vi "Shot Info Collection.vi"(6 "Vision Target Aligned? in":bool, 7 "Current Angle":dbl, 8 "Reinit?":bool, 9 "Shot Type":T1, 10 "Vision Packet":T2, 11 "Shooter Presets":T3={"Batter Shot"={"L"=0.0, "R"=0.0, "A"=0.0}, "Deep Middle"={"L"=0.0, "R"=0.0, "A"=0.0}, "Manual Shot"={"L"=0.0, "R"=0.0, "A"=0.0}, "Left Ticks Per Rotation"=0.0, "Right Ticks Per Rotation"=0.0, "Low Bar Shot"={"L"=0.0, "R"=0.0, "A"=0.0}, "Shooter RPM Tolerance"=0.0, "Trigger Power"=0.0, "Fire from Load Delay"=0, "Max Angle"=0.0, "Min Angle"=0.0, "Angle PID gains"={"P"=0.0, "I"=0.0, "D"=0.0}, "Angle Output"={"output high"=0.0, "output low"=0.0}, "Shooter Angle Tolerance"=0.0, "Vision Shoot x^2"=0.0, "Vision Shoot x"=0.0, "Feed Forward Max Accel"=0.0, "Feed Forward Kv"=0.0, "Backwards Trigger"=0.0, "Shot Finish Delay (ms)"=0.0, "Angle Max Current"=0.0, "Angle Current Trip Time"=0.0, "Intake Angle"=0.0, "Vision Shoot c"=0.0, "Reset?"=FALSE, "Button Release Delay"=0.0, "Angle Pot x"=0.0, "Angle Pot c"=0.0, "Ignore Angle?"=FALSE, "Max RPM"=0.0, "Safty Frist Angle"=0.0, "Intake Danger Height"=0.0, "Angle Pot B"=0, "Angle Pot M"=0.0, "FF Finish RPM"=0.0, "RPM PID Right"={"P"=1.0, "I"=0.01, "D"=0.0, "FF"=0.0}, "RPM PID Left"={"P"=1.0, "I"=0.01, "D"=0.0, "FF"=0.0}, "Backwards RPM"=0.0, "Vision RPM"=0.0, "Run Wheels Backward Delay"=0, "Cleat Shot"={"L"=0.0, "R"=0.0, "A"=0.0}, "Vision Far RPM"=0.0, "Vision Far Distance"=0.0, "Vision Far Angle"=0.0}) -> (2 "Right Wheel RPM":dbl, 3 "Left Wheel RPM":dbl, 4 "Angle":dbl, 5 "Vision Target Aligned? out":bool)   [LabVIEW 2015]
uses:
  Common Code/Shooter Presets.ctl
  Common Code/Shot Presets.ctl
  Common Code/Goal Vision Packet.ctl
  Common Code/Shot Type.ctl
  Common Code/Change Detect Int.vi
  Common Code/Change Detect Boolean.vi
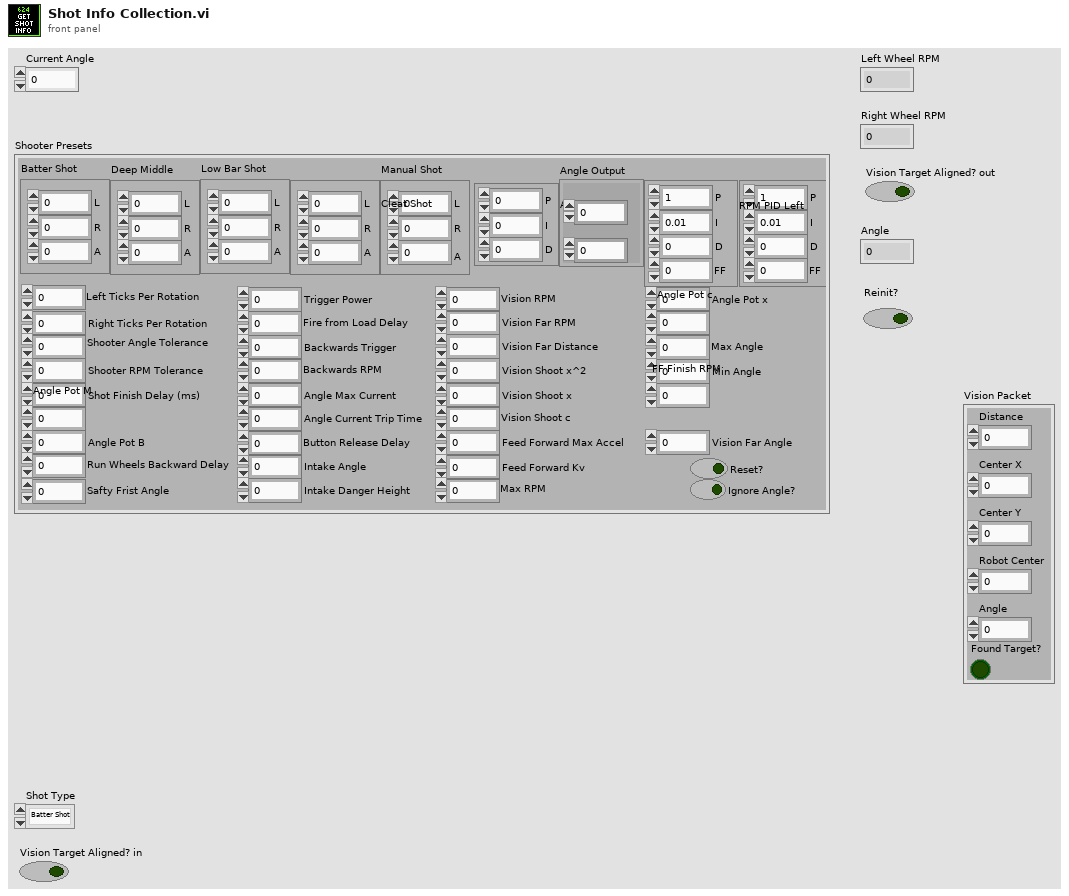
[diagram p1: front panel]
types:
  T1 = typedef "Shot Type.ctl" = enum16{"Batter Shot", "Corner Shot", "Cleat Shot", "Vision Shot", "Deep Middle Shot"}
  T2 = typedef "Goal Vision Packet.ctl" = cluster{"Distance":dbl, "Center X":dbl, "Center Y":dbl, "Found Target?":bool, "Robot Center":dbl, "Angle":dbl}
  T3 = typedef "Shooter Presets.ctl" = cluster{"Batter Shot":T4, "Deep Middle":T4, "Manual Shot":T4, "Left Ticks Per Rotation":dbl, "Right Ticks Per Rotation":dbl, "Low Bar Shot":T4, "Shooter RPM Tolerance":dbl, "Trigger Power":dbl, "Fire from Load Delay":i32, "Max Angle":dbl, "Min Angle":dbl, "Angle PID gains":cluster{"P":dbl, "I":dbl, "D":dbl}, "Angle Output":cluster{"output high":dbl, "output low":dbl}, "Shooter Angle Tolerance":dbl, "Vision Shoot x^2":dbl, "Vision Shoot x":dbl, "Feed Forward Max Accel":dbl, "Feed Forward Kv":dbl, "Backwards Trigger":dbl, "Shot Finish Delay (ms)":dbl, "Angle Max Current":dbl, "Angle Current Trip Time":dbl, "Intake Angle":dbl, "Vision Shoot c":dbl, "Reset?":bool, "Button Release Delay":dbl, "Angle Pot x":dbl, "Angle Pot c":dbl, "Ignore Angle?":bool, "Max RPM":dbl, "Safty Frist Angle":dbl, "Intake Danger Height":dbl, "Angle Pot B":i32, "Angle Pot M":dbl, "FF Finish RPM":dbl, "RPM PID Right":cluster{"P":dbl, "I":dbl, "D":dbl, "FF":dbl}, "RPM PID Left":cluster{"P":dbl, "I":dbl, "D":dbl, "FF":dbl}, "Backwards RPM":dbl, "Vision RPM":dbl, "Run Wheels Backward Delay":u32, "Cleat Shot":T4, "Vision Far RPM":dbl, "Vision Far Distance":dbl, "Vision Far Angle":dbl}
  T4 = typedef "Shot Presets.ctl" = cluster{"L":dbl, "R":dbl, "A":dbl}
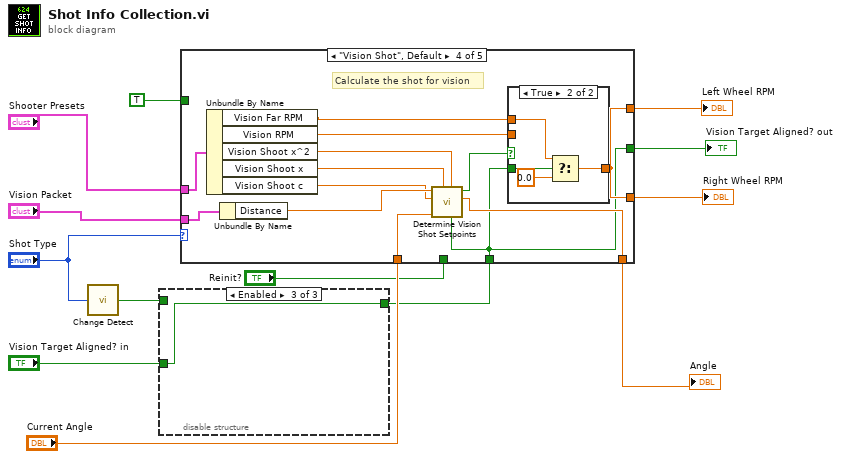
[diagram p0: block diagram]
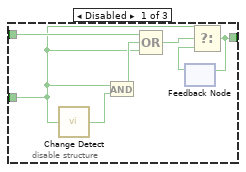
[diagram p2: hidden frame]
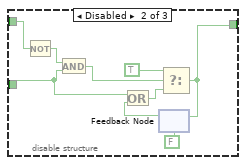
[diagram p3: hidden frame]
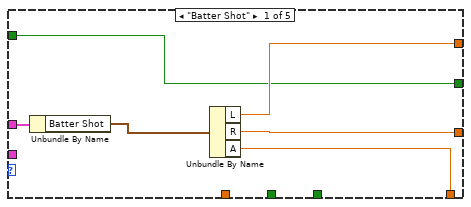
[diagram p4: hidden frame]
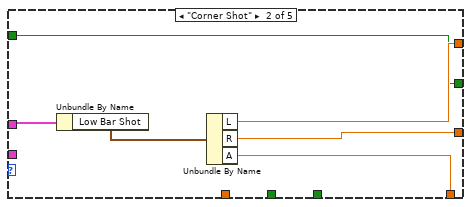
[diagram p5: hidden frame]
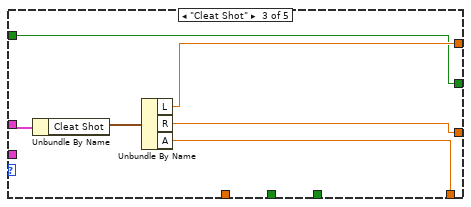
[diagram p6: hidden frame]
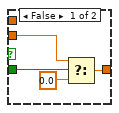
[diagram p7: hidden frame]
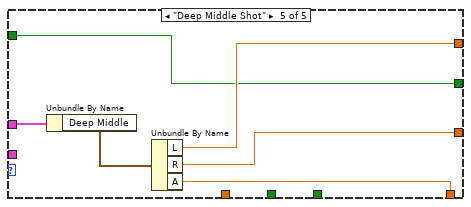
[diagram p8: hidden frame]
diagram:
  n1 = call-poly "Change Detect.vi"("In"="Shot Type") -> ("Changed?"=w4:bool)
  n2 = disable-structure shown="Enabled" {
    disable-tunnel: w4 -> [w20 w26 _]
    disable-tunnel: [w18 w24 w30] -> w3
    disable-tunnel: "Vision Target Aligned? in" -> [w14 w22 w30]
    frame Disabled {
      n3 = call-poly "Change Detect.vi"("In"=w14) -> ("Changed?"=w16:bool)
      n4 = And(x=w14, y=w16) -> (x .and. y?=w15:bool)
      n5 = Compound Arithmetic op=OR(w20, w15, w14) -> (w19:bool)
      n6 = feedback #1() -> (w17:bool)  [unwired: 1 in]
      n7 = Select(t=w14, s=w19, f=w17) -> (s? t:f=w18:bool)
      n8 = feedback-in #1(w18) -> ()
    }
    frame Disabled {
      n9 = Not(x=w26) -> (.not. x?=w25:bool)
      n10 = And(x=w25, y=w22) -> (x .and. y?=w27:bool)
      n11 = feedback #2(FALSE) -> (w23:bool)
      n12 = Or(x=w22, y=w23) -> (x .or. y?=w21:bool)
      n13 = Select(t=TRUE, s=w27, f=w21) -> (s? t:f=w24:bool)
      n14 = feedback-in #2(w24) -> ()
    }
    frame Enabled {
    }
  }
  n15 = case shown="\"Vision Shot\", Default" "Shot Type" {
    tunnel: "Shooter Presets" -> [w36 w42 w48 w61 w75]
    tunnel: [w34 w38 w46 w53 w73] -> w6
    tunnel: [w33 w39 w45 w53 w72] -> w7
    tunnel: "Vision Packet" -> [_ _ _ w59 _]
    tunnel: [w32 w37 w43 w52 w71] -> w9
    tunnel: w3 -> [_ _ _ w52 _]
    tunnel: TRUE -> [w32 w37 w43 _ w71]
    tunnel: [w31 w40 w44 w58 w70] -> w11
    tunnel: "Current Angle" -> [_ _ _ w51 _]
    tunnel: "Reinit?" -> [_ _ _ _ _]
    frame "Batter Shot" {
      n16 = Unbundle By Name(w36) -> ("Batter Shot"=w35:T4)
      n17 = Unbundle By Name(w35) -> ("L"=w34:dbl, "R"=w33:dbl, "A"=w31:dbl)
    }
    frame "Corner Shot" {
      n18 = Unbundle By Name(w42) -> ("Low Bar Shot"=w41:T4)
      n19 = Unbundle By Name(w41) -> ("L"=w38:dbl, "R"=w39:dbl, "A"=w40:dbl)
    }
    frame "Cleat Shot" {
      n20 = Unbundle By Name(w48) -> ("Cleat Shot"=w47:T4)
      n21 = Unbundle By Name(w47) -> ("L"=w46:dbl, "R"=w45:dbl, "A"=w44:dbl)
    }
    frame "Vision Shot", Default {
      # "Calculate the shot for vision"
      n22 = Unbundle By Name(w61) -> ("Vision Far RPM"=w50:dbl, "Vision RPM"=w54:dbl, "Vision Shoot x^2"=w56:dbl, "Vision Shoot x"=w57:dbl, "Vision Shoot c"=w55:dbl)
      n23 = Unbundle By Name(w59) -> ("Distance"=w60:dbl)
      n24 = call "Determine Vision Shot Setpoints.vi"("Vision Aligned?"=w52, "x^2"=w56, "x"=w57, "Current Angle"=w51, "c"=w55, "Distance from Target"=w60) -> ("Angle"=w58:dbl, "Are We really far aWaY?"=w49:bool)  [unwired: 4 in]
      n25 = case shown="True" w49 {
        tunnel: w54 -> [w65 _]
        tunnel: [w63 w66] -> w53
        tunnel: w52 -> [w62 w69]
        tunnel: w50 -> [_ w68]
        frame False {
          n26 = Select(t=w65, s=w62, f=0.0) -> (s? t:f=w63:dbl)
        }
        frame True {
          n27 = Select(t=w68, s=w69, f=0.0) -> (s? t:f=w66:dbl)
        }
      }
    }
    frame "Deep Middle Shot" {
      n28 = Unbundle By Name(w75) -> ("Deep Middle"=w74:T4)
      n29 = Unbundle By Name(w74) -> ("L"=w73:dbl, "R"=w72:dbl, "A"=w70:dbl)
    }
  }
  "Angle" <- w11
  "Vision Target Aligned? out" <- w9
  "Right Wheel RPM" <- w7
  "Left Wheel RPM" <- w6
